vi "Read Message.vi"(8 "error in":errorcluster, 9 "MaxRead":i32, 10 "ID":u32, 11 "Channel in":u16) -> (0 "error out":errorcluster, 1 "Passed":bool, 2 "Last Message":T1, 3 "Channel out":u16, 4 "Negative":bool)   [LabVIEW 2023]
uses:
  PCAN2023/PCAN API.lvlib
  <vilib>/Utility/file.llb/Write Delimited Spreadsheet (string).vi
panel:
  out "MessageBuffer out 3":T1 {"ID" format="%.0x"; "DATA[0]" format="%.0x"; "DATA[1]" format="%.0x"; "DATA[2]" format="%.0x"; "DATA[3]" format="%.0x"; "DATA[4]" format="%.0x"; "DATA[5]" format="%.0x"; "DATA[6]" format="%.0x"; "DATA[7]" format="%.0x"}
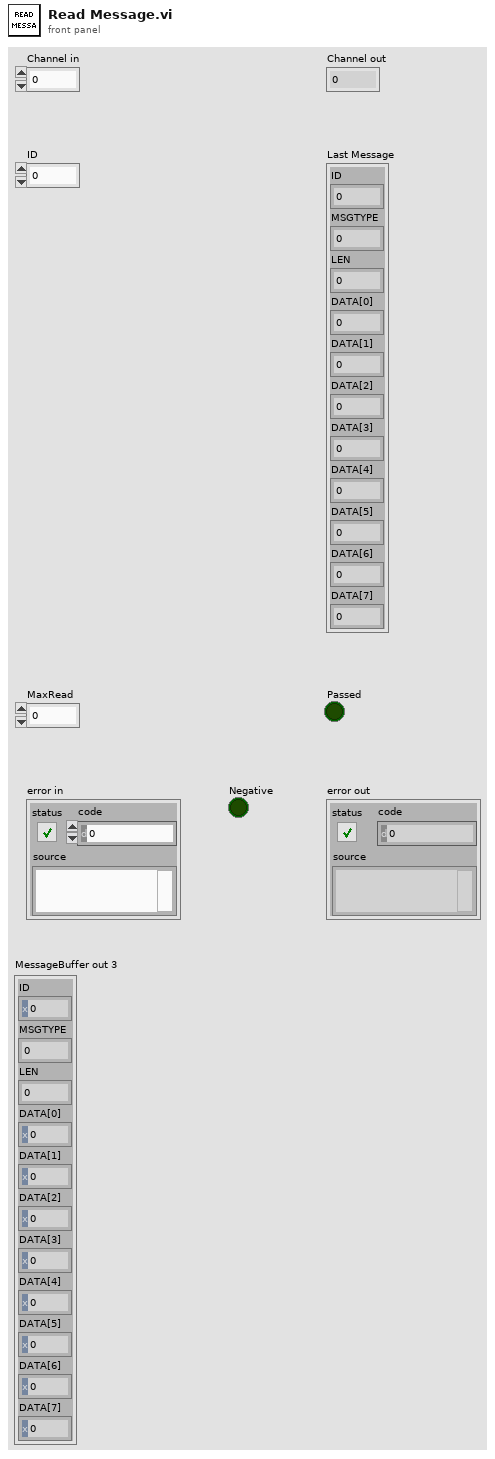
[diagram p1: front panel]
types:
  T1 = cluster{"ID":u32, "MSGTYPE":u8, "LEN":u8, "DATA[0]":u8, "DATA[1]":u8, "DATA[2]":u8, "DATA[3]":u8, "DATA[4]":u8, "DATA[5]":u8, "DATA[6]":u8, "DATA[7]":u8}
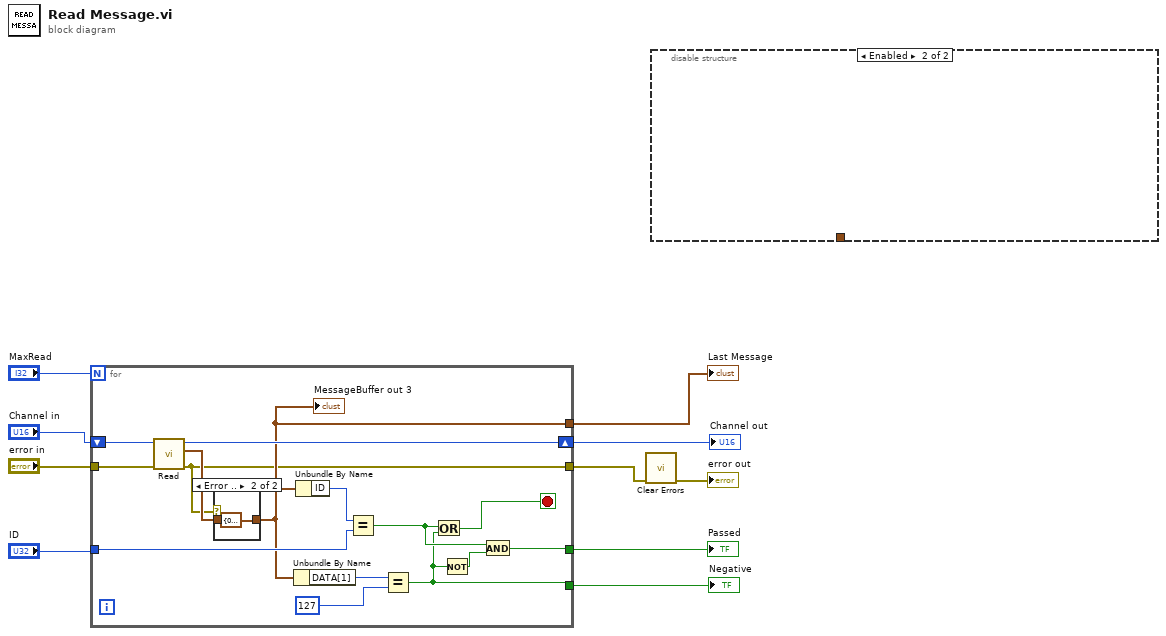
[diagram p0: block diagram]
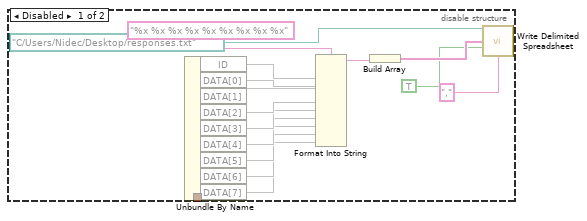
[diagram p2: hidden frame]
diagram:
  n1 = for {
    N: "MaxRead" -> [_]
    shift-right: [w24] -> w7
    shift-left: "Channel in" -> [w25]
    tunnel: "ID" -> [w22]
    tunnel: [w13] -> w3
    tunnel: [w12] -> w2
    tunnel: "error in" -> [w21]
    tunnel: [w15] -> w6
    tunnel: [w17] -> w5
    stop <- w11 stop-if-true
    n2 = call "Read.vi"("error in"=w21, "Channel"=w25) -> ("error out"=w12:errorcluster, "MessageBuffer out"=w14:T1, "Channel out"=w24:u16)  [unwired: 6 in, 1 out]
    n3 = case shown="Error .." w12 {
      tunnel: w14 -> [w26 _]
      tunnel: [w26 T1 {"ID"=0, "MSGTYPE"=0, "LEN"=0, "DATA[0]"=0, "DATA[1]"=127, "DATA[2]"=0, "DATA[3]"=0, "DATA[4]"=0, "DATA[5]"=0, "DATA[6]"=0, "DATA[7]"=0}] -> w13
      frame No Error {
      }
      frame Error {
      }
    }
    "MessageBuffer out 3" <- w13
    n4 = Unbundle By Name(w13) -> ("DATA[1]"=w20:u8)
    n5 = Unbundle By Name(w13) -> ("ID"=w23:u32)
    n6 = Equal?(x=w23, y=w22) -> (x = y?=w18:bool)
    n7 = Equal?(x=w20, y=u8 127) -> (x = y?=w17:bool)
    n8 = Or(x=w18, y=w17) -> (x .or. y?=w11:bool)
    n9 = Not(x=w17) -> (.not. x?=w16:bool)
    n10 = And(x=w18, y=w16) -> (x .and. y?=w15:bool)
  }
  "Last Message" <- w3
  "Channel out" <- w7
  "Passed" <- w6
  "Negative" <- w5
  n11 = call <vilib>:"Clear Errors.vi"("error in (no error)"=w2) -> ("error out"=→"error out":errorcluster)  [unwired: 5 in, 1 out]
  n12 = disable-structure shown="Enabled" {
    disable-tunnel: _ -> [w42 _]
    frame Disabled {
      n13 = Unbundle By Name(w42) -> ("ID"=w41, "DATA[0]"=w35, "DATA[1]"=w34, "DATA[2]"=w33, "DATA[3]"=w32, "DATA[4]"=w31, "DATA[5]"=w30, "DATA[6]"=w29, "DATA[7]"=w28)
      n14 = Format Into String(format string="%x %x %x %x %x %x %x %x %x", w41, w35, w34, w33, w32, w31, w30, w29, w28) -> (resulting string=w40:string)  [unwired: 2 in, 1 out]
      n15 = Build Array(w40) -> (w39:string[])
      n16 = call-poly <vilib>:"Write Delimited Spreadsheet.vi"("file path (dialog if empty)"=path "C:/Users/Nidec/Desktop/responses.txt", "1D data"=w39, "append to file? (new file:F)"=TRUE, "delimiter (\\t)"="," ("delimiter (\\t)")) -> ()  [unwired: 10 in, 2 out]
    }
    frame Enabled {
    }
  }
